vi "UDT_application_Set Data Out.vi"() -> (3 "Unit Test Framework Results":T1)   [LabVIEW 2017]
doc: "Use this template to create a user-defined test VI. Define your test requirements and wire the results to the <b>Result (Test)</b> control. Do not modify the <b>Unit Test Framework Results</b> indicator."
uses:
  <vilib>/utf/common/utf_test_result_troll.ctl
  <vilib>/utf/common/utf_test_result.ctl
  <vilib>/utf/common/utf_test_result_failure.ctl
  <vilib>/utf/common/utf_test_comparison_operators.ctl
  <vilib>/utf/common/utf_vi_tag.ctl
  RT/TypeDefs/dataOut.ctl
  RT/SubVIs/FGVs/TypeDefs/DataFGVControl.ctl
  <vilib>/Control Software Solutions Ltd/UTF Helper/SubVIs/UTF Boolean Equals.vi
  <vilib>/Control Software Solutions Ltd/UTF Helper/SubVIs/UTF Double Equals.vi
  <vilib>/Control Software Solutions Ltd/UTF Helper/SubVIs/UTF I32 Equals.vi
  <vilib>/Control Software Solutions Ltd/UTF Helper/Unit Test Helper.lvlib
  <vilib>/utf/NI_UnitTestFramework.lvlib
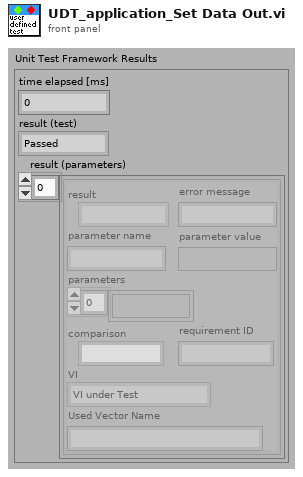
[diagram p1: front panel]
types:
  T1 = typedef "NI_UnitTestFramework.lvlib/utf_test_result_troll.ctl" = cluster{"time elapsed [ms]":u32, "result (test)":T2, "result (parameters)":T3[]}
  T2 = typedef "NI_UnitTestFramework.lvlib/utf_test_result.ctl" = enum16{"Passed", "Failed", "Error", "Skipped", "Not Processed"}
  T3 = typedef "NI_UnitTestFramework.lvlib/utf_test_result_failure.ctl" = cluster{"result":T2, "error message":string, "parameter name":string, "parameter value":variant, "parameters":variant[], "comparison":T4, "requirement ID":string, "VI":T5, "Used Vector Name":string}
  T4 = typedef "NI_UnitTestFramework.lvlib/utf_test_comparison_operators.ctl" = enum16{"=", "!=", ">", ">=", "<", "<=", "range", "symmetric tolerance", "asymmetric tolerance", "string contains", "string not contain", "array size", "string length", "array range", "by element", "array range (limit array)", "user-defined", "array contains", "array not contain", "vector length", "= (elm)", "!= (elm)", "= (case insensitive)", "!= (case insensitive)"}
  T5 = typedef "NI_UnitTestFramework.lvlib/utf_vi_tag.ctl" = enum16{"Setup VI", "VI under Test", "Teardown VI"}
  T6 = typedef "DataFGVControl.ctl" = enum16{"Set Data", "Get Data"}
  T7 = typedef "dataOut.ctl" = cluster{"X0pos":dbl, "Y0pos":dbl, "Z0pos":dbl, "Fx":dbl, "Fy":dbl, "Fz":dbl, "Encoder1":i32, "Encoder2":i32, "Pot1":dbl, "Pot2":dbl, "Theta0":dbl, "Theta1":dbl, "X1pos":dbl, "Y1pos":dbl, "Z1pos":dbl, "X2pos":dbl, "Y2pos":dbl, "Z2pos":dbl, "ErrorOccurred":bool}
  T8 = typedef "allData.ctl" = cluster{"DataOut":T7, "DataIn":T9}
  T9 = typedef "dataIn.ctl" = cluster{"Xtarget":dbl, "Ytarget":dbl, "Ztarget":dbl, "X_Attractor 1":dbl, "Y_Attractor 1":dbl, "Z_Attractor 1":dbl, "X_Attractor 2":dbl, "Y_Attractor 2":dbl, "Z_Attractor 2":dbl, "Traj Flag":bool, "DeadZone":dbl, "Assistance":bool, "Shutdown?":bool, "AssistanceLevel":dbl}
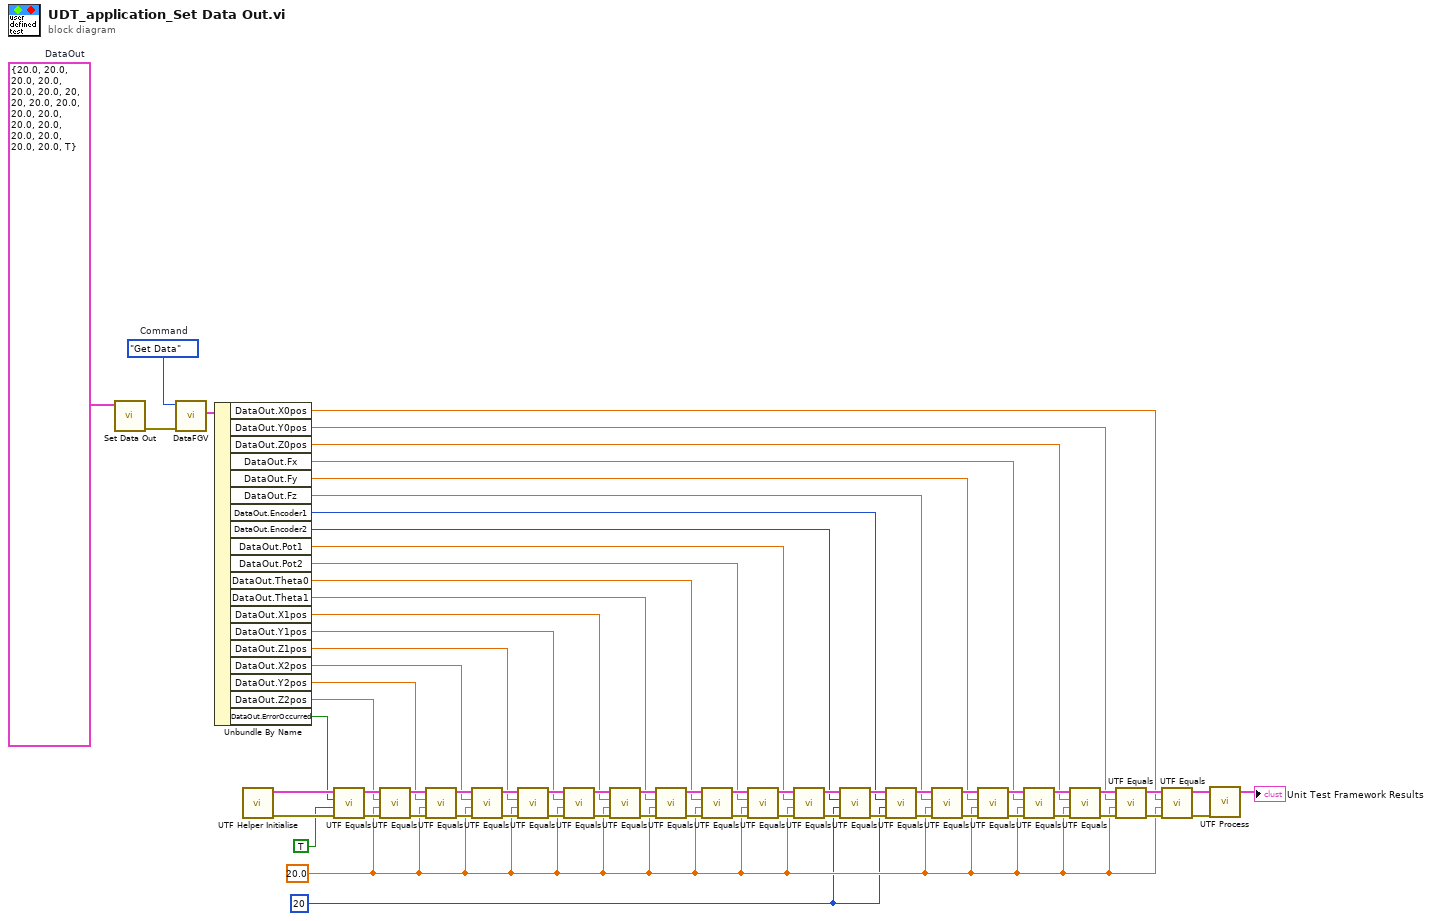
[diagram p0: block diagram]
diagram:
  w1 = 20 ("Encoder2")
  w2 = 20.0 ("Z2pos")
  w66 = DataFGVControl."Get Data"  # Command
  w67 = T7 {"X0pos"=20.0, "Y0pos"=20.0, "Z0pos"=20.0, "Fx"=20.0, "Fy"=20.0, "Fz"=20.0, "Encoder1"=20, "Encoder2"=20, "Pot1"=20.0, "Pot2"=20.0, "Theta0"=20.0, "Theta1"=20.0, "X1pos"=20.0, "Y1pos"=20.0, "Z1pos"=20.0, "X2pos"=20.0, "Y2pos"=20.0, "Z2pos"=20.0, "ErrorOccurred"=TRUE}  # DataOut
  n1 = call "Set Data Out.vi"("DataOut"=w67) -> ("error out"=w65:errorcluster)  [unwired: 10 in]
  n2 = call "DataFGV.vi"("error in (no error)"=w65, "Command"=w66) -> ("AllData out"=w64:T8)  [unwired: 8 in, 1 out]
  n3 = Unbundle By Name(w64) -> ("DataOut.X0pos"=w7:dbl, "DataOut.Y0pos"=w10:dbl, "DataOut.Z0pos"=w11:dbl, "DataOut.Fx"=w12:dbl, "DataOut.Fy"=w13:dbl, "DataOut.Fz"=w14:dbl, "DataOut.Encoder1"=w15:i32, "DataOut.Encoder2"=w16:i32, "DataOut.Pot1"=w17:dbl, "DataOut.Pot2"=w18:dbl, "DataOut.Theta0"=w19:dbl, "DataOut.Theta1"=w20:dbl, "DataOut.X1pos"=w22:dbl, "DataOut.Y1pos"=w23:dbl, "DataOut.Z1pos"=w24:dbl, "DataOut.X2pos"=w25:dbl, "DataOut.Y2pos"=w26:dbl, "DataOut.Z2pos"=w27:dbl, "DataOut.ErrorOccurred"=w61:bool)
  n4 = call <vilib>:"UTF Helper Initialise.vi"() -> ("error out"=w62:errorcluster, "results array"=w63:T3[])  [unwired: 10 in]
  n5 = call-poly <vilib>:"UTF Equals.vi"("error in (no error)"=w62, "Test Value"=TRUE, "Input"=w61, "Input Results"=w63) -> ("error out"=w60:errorcluster, "Output Results"=w59:T3[])  [unwired: 6 in]
  n6 = call-poly <vilib>:"UTF Equals.vi"("error in (no error)"=w60, "Test Value"=w2, "Input"=w27, "Input Results"=w59) -> ("error out"=w58:errorcluster, "Output Results"=w57:T3[])  [unwired: 6 in]
  n7 = call-poly <vilib>:"UTF Equals.vi"("error in (no error)"=w58, "Test Value"=w2, "Input"=w26, "Input Results"=w57) -> ("error out"=w56:errorcluster, "Output Results"=w55:T3[])  [unwired: 6 in]
  n8 = call-poly <vilib>:"UTF Equals.vi"("error in (no error)"=w56, "Test Value"=w2, "Input"=w25, "Input Results"=w55) -> ("error out"=w54:errorcluster, "Output Results"=w53:T3[])  [unwired: 6 in]
  n9 = call-poly <vilib>:"UTF Equals.vi"("error in (no error)"=w54, "Test Value"=w2, "Input"=w24, "Input Results"=w53) -> ("error out"=w52:errorcluster, "Output Results"=w51:T3[])  [unwired: 6 in]
  n10 = call-poly <vilib>:"UTF Equals.vi"("error in (no error)"=w52, "Test Value"=w2, "Input"=w23, "Input Results"=w51) -> ("error out"=w21:errorcluster, "Output Results"=w39:T3[])  [unwired: 6 in]
  n11 = call-poly <vilib>:"UTF Equals.vi"("error in (no error)"=w21, "Test Value"=w2, "Input"=w22, "Input Results"=w39) -> ("error out"=w46:errorcluster, "Output Results"=w45:T3[])  [unwired: 6 in]
  n12 = call-poly <vilib>:"UTF Equals.vi"("error in (no error)"=w46, "Test Value"=w2, "Input"=w20, "Input Results"=w45) -> ("error out"=w47:errorcluster, "Output Results"=w40:T3[])  [unwired: 6 in]
  n13 = call-poly <vilib>:"UTF Equals.vi"("error in (no error)"=w47, "Test Value"=w2, "Input"=w19, "Input Results"=w40) -> ("error out"=w48:errorcluster, "Output Results"=w38:T3[])  [unwired: 6 in]
  n14 = call-poly <vilib>:"UTF Equals.vi"("error in (no error)"=w48, "Test Value"=w2, "Input"=w18, "Input Results"=w38) -> ("error out"=w49:errorcluster, "Output Results"=w37:T3[])  [unwired: 6 in]
  n15 = call-poly <vilib>:"UTF Equals.vi"("error in (no error)"=w49, "Test Value"=w2, "Input"=w17, "Input Results"=w37) -> ("error out"=w50:errorcluster, "Output Results"=w36:T3[])  [unwired: 6 in]
  n16 = call-poly <vilib>:"UTF Equals.vi"("error in (no error)"=w50, "Test Value"=w1, "Input"=w16, "Input Results"=w36) -> ("error out"=w28:errorcluster, "Output Results"=w29:T3[])  [unwired: 6 in]
  n17 = call-poly <vilib>:"UTF Equals.vi"("error in (no error)"=w28, "Test Value"=w1, "Input"=w15, "Input Results"=w29) -> ("error out"=w44:errorcluster, "Output Results"=w35:T3[])  [unwired: 6 in]
  n18 = call-poly <vilib>:"UTF Equals.vi"("error in (no error)"=w44, "Test Value"=w2, "Input"=w14, "Input Results"=w35) -> ("error out"=w43:errorcluster, "Output Results"=w34:T3[])  [unwired: 6 in]
  n19 = call-poly <vilib>:"UTF Equals.vi"("error in (no error)"=w43, "Test Value"=w2, "Input"=w13, "Input Results"=w34) -> ("error out"=w42:errorcluster, "Output Results"=w33:T3[])  [unwired: 6 in]
  n20 = call-poly <vilib>:"UTF Equals.vi"("error in (no error)"=w42, "Test Value"=w2, "Input"=w12, "Input Results"=w33) -> ("error out"=w41:errorcluster, "Output Results"=w32:T3[])  [unwired: 6 in]
  n21 = call-poly <vilib>:"UTF Equals.vi"("error in (no error)"=w41, "Test Value"=w2, "Input"=w11, "Input Results"=w32) -> ("error out"=w30:errorcluster, "Output Results"=w31:T3[])  [unwired: 6 in]
  n22 = call-poly <vilib>:"UTF Equals.vi"("error in (no error)"=w30, "Test Value"=w2, "Input"=w10, "Input Results"=w31) -> ("error out"=w9:errorcluster, "Output Results"=w8:T3[])  [unwired: 6 in]
  n23 = call-poly <vilib>:"UTF Equals.vi"("error in (no error)"=w9, "Test Value"=w2, "Input"=w7, "Input Results"=w8) -> ("error out"=w6:errorcluster, "Output Results"=w5:T3[])  [unwired: 6 in]
  n24 = call <vilib>:"UTF Process.vi"("error in (no error)"=w6, "results array"=w5) -> ("Unit Test Framework Results"=→"Unit Test Framework Results":T1)  [unwired: 9 in]
